vi "Confocal_0823.vi"() -> ()   [LabVIEW 2017]
uses:
  <vilib>/Math Plots/2D Math Plots/XY Plot Matrix/XY Plot Matrix XCtrl/XY Plot Matrix.xctl
  Public/Documents/SIToolkit/LabVIEW/ExamplesXX_4_3_1_4/Spectroscopy Applications/GlobalCamOpen.vi
  Public/Documents/SIToolkit/LabVIEW/ExamplesXX_4_3_1_4/Spectroscopy Applications/GlobalInitializeFlag.vi
  Public/Documents/SIToolkit/LabVIEW/ExamplesXX_4_3_1_4/Spectroscopy Applications/GlobalTimingMode.vi
  Public/Documents/SIToolkit/LabVIEW/ExamplesXX_4_3_1_4/Spectroscopy Applications/GlobalFramesToStr.vi
  Public/Documents/SIToolkit/LabVIEW/ExamplesXX_4_3_1_4/Spectroscopy Applications/GlobalAcquireFocusFlag.vi
  Public/Documents/SIToolkit/LabVIEW/ExamplesXX_4_3_1_4/Spectroscopy Applications/GlobalExposure.vi
  <vilib>/Math Plots/2D Math Plots/XY Plot Matrix/XY Plot Matrix Datatype/XY Plot Matrix Datatype.lvclass
panel:
  out "Position 7":dbl[](array[numeric]) format="%.6f"
  out "Position 4":dbl[](array[numeric]) format="%.6f"
  in  "error PI Stage":errorcluster
  out "error out 2":errorcluster
  in  "Tab Control":T1(tab)
  in  "Focus/Acquire Mode":u32=1 min=1 max=5 step=1
  in  "Number of Frames to store":u32=1 min=1 step=1
  in  "Timing Mode":u32(ring)=1 items=["N/A", "Free Run/Timed", "Trigger First (PM only)", "Ext Sync/Strobed ", "Variable Exp (PM only)", "Flash Mode (PM only)"]
  out "Pixel Time":i32
  out "Bit Depth":i32
  out "ReadOut port":i32
  out "ADC Speed":i32
  in  "Set Experiment \nParameters, Initialize \nCamera/Controller":bool
  out "Read Temp.":dbl format="%.2f"
  in  "Set Temp.":dbl format="%.2f"
  in  "Exposure 2":dbl=0.2 format="%.2f"
  out "Controller Initialized":bool
  in  "error in":errorcluster
  out "error out":errorcluster
  in  "Power":dbl=10.0
  in  "Frequency":dbl=2810.0
  in  "Release Camera":bool
  out "Position 6":dbl[](array[numeric]) format="%.6f"
  out "Conn. Axis 5":string[](array[string])
  out "error out 3":errorcluster
  out "COM Error":bool
  out "Camera Opened":bool
  in  "Number of Steps Left":dbl=5.0 format="%#_13g"
  in  "OK Button 5":bool
  in  "Step Size (microns)":dbl[](array[numeric])=[0.01]
  out "XY Plot Matrix":refnum<class "XY Plot Matrix Datatype.lvclass">[](xcontrol)
  in  "Number of Steps Down":dbl=5.0 format="%#_13g"
  out "Position":dbl[](array[numeric]) format="%.6f"
  out "Position 3":dbl[](array[numeric]) format="%.6f"
  in  "stop 2":bool
  out "Line Number":i32
  out "Position 2":dbl[](array[numeric]) format="%.6f"
  in  "?":bool
  out "Position 5":dbl[](array[numeric]) format="%.6f"
  in  "Step Size (microns) Y":dbl[](array[numeric])=[0.01]
  in  "Step Size (microns) X":dbl[](array[numeric])=[0.01]
  out "Position 8":dbl[](array[numeric]) format="%.6f"
  in  "?":bool
  out "Acquire Graph":sgl[](graph)
  out "Collecting Data":bool
  in  "Full File Name for Acqure":path
  in  "OK Button":bool
  # "The following are read \nfrom camera after setting\nvalues to left.\n-1 value means item is not \nsupported by camera."
  # "Stage position on connection."
  # "Be sure to put in a full file name below before starting."
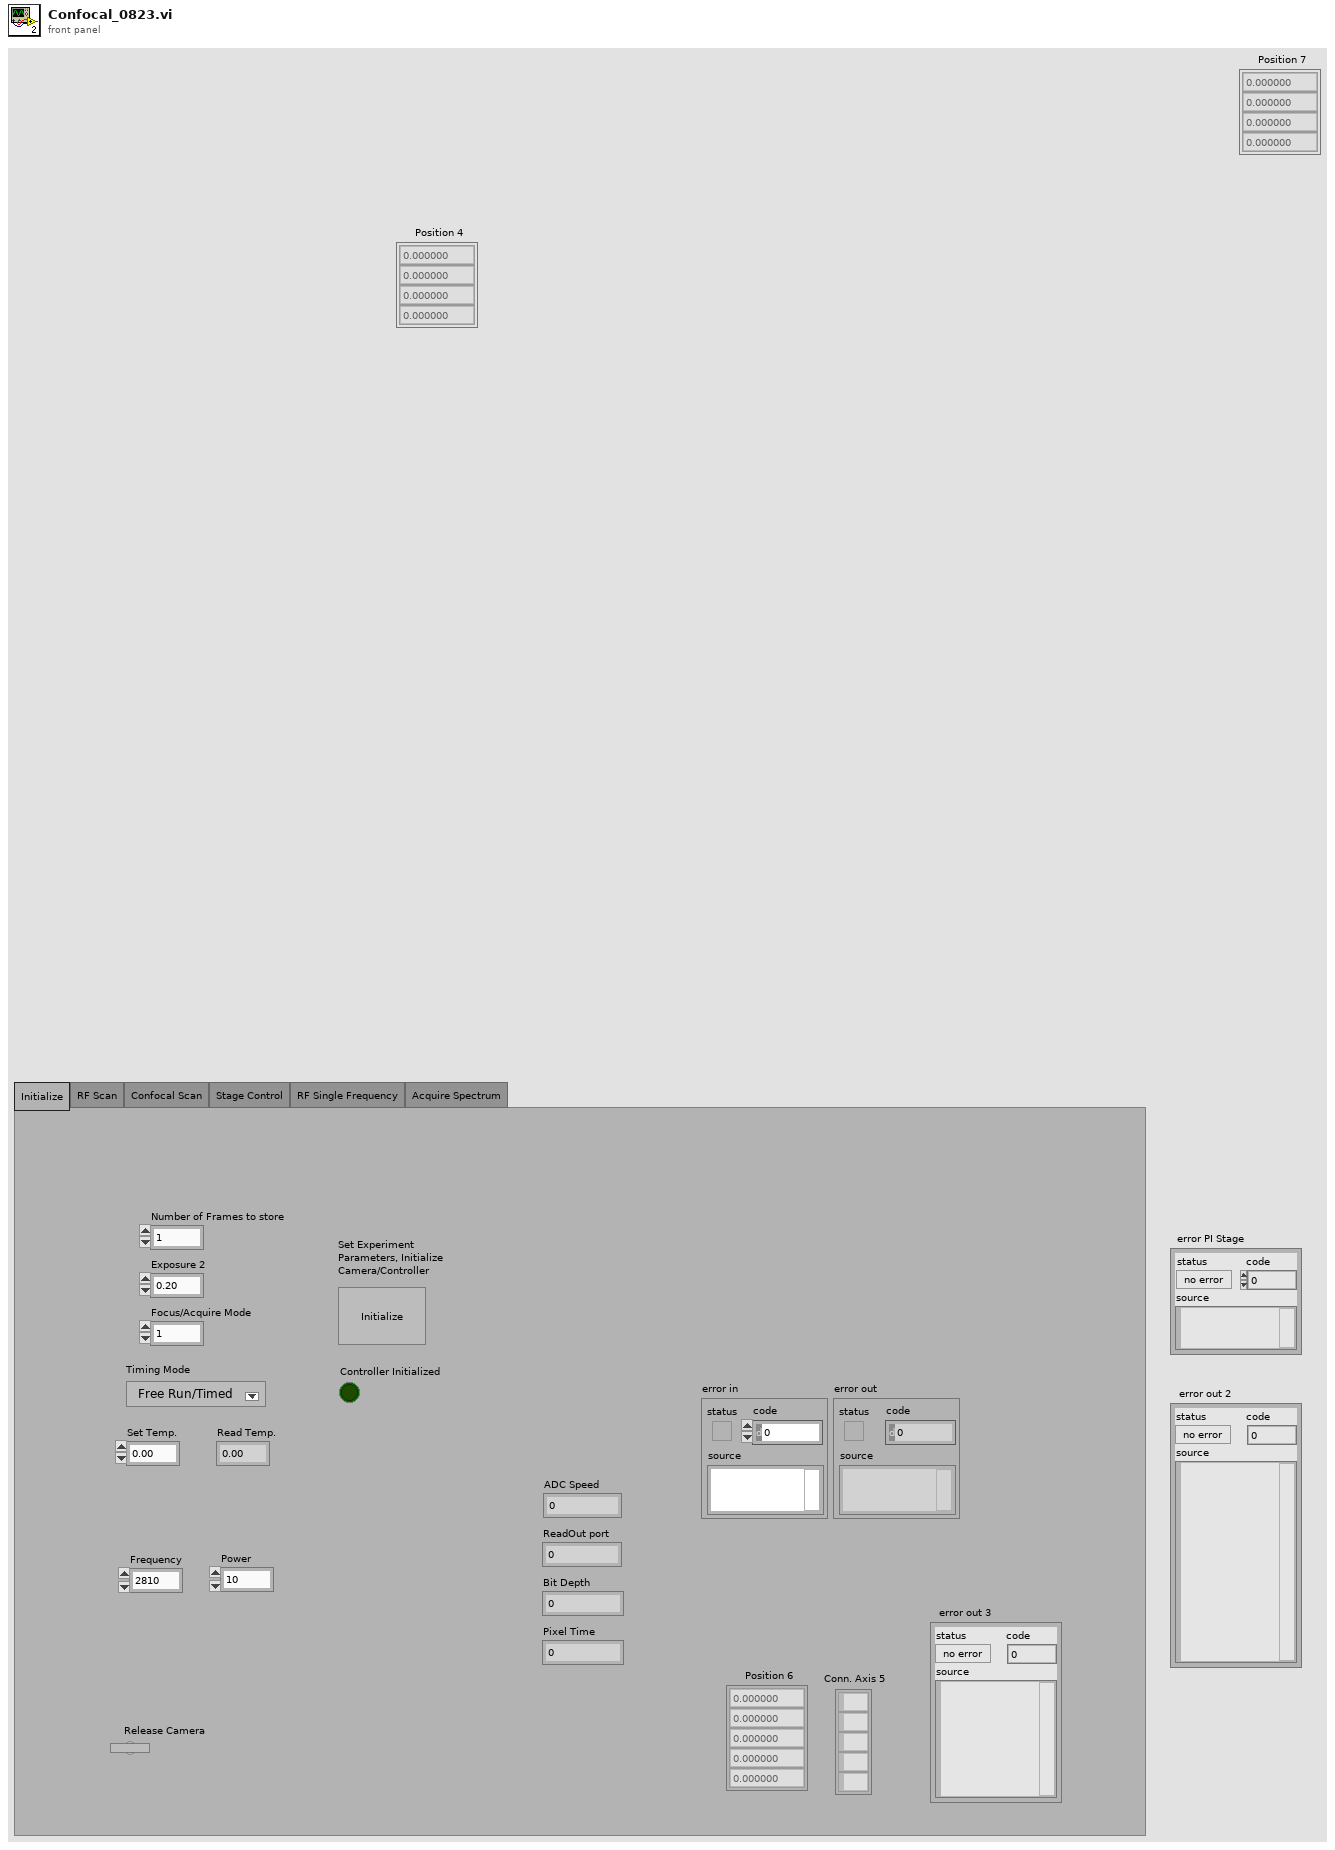
[diagram p1: front panel]
types:
  T1 = enum32{"Initialize", "RF Scan", "Confocal Scan", "Stage Control", "RF Single Frequency", "Acquire Spectrum"}
  T2 = cluster{"X start":u32, "X end":u32, "X Binning/Grouping":u32, "Y start":u32, "Y end":u32, "Y Binning/Grouping":u32}
  T3 = cluster{"Host address/name":string, "Port":i32, "Board":i32, "TCP/IP Search?":bool}
  T4 = cluster{"Camera Handle":u32, "Pulser Handle":u32, "File Handle":u32, "Display Handle":u32, "Image Handle":u32}
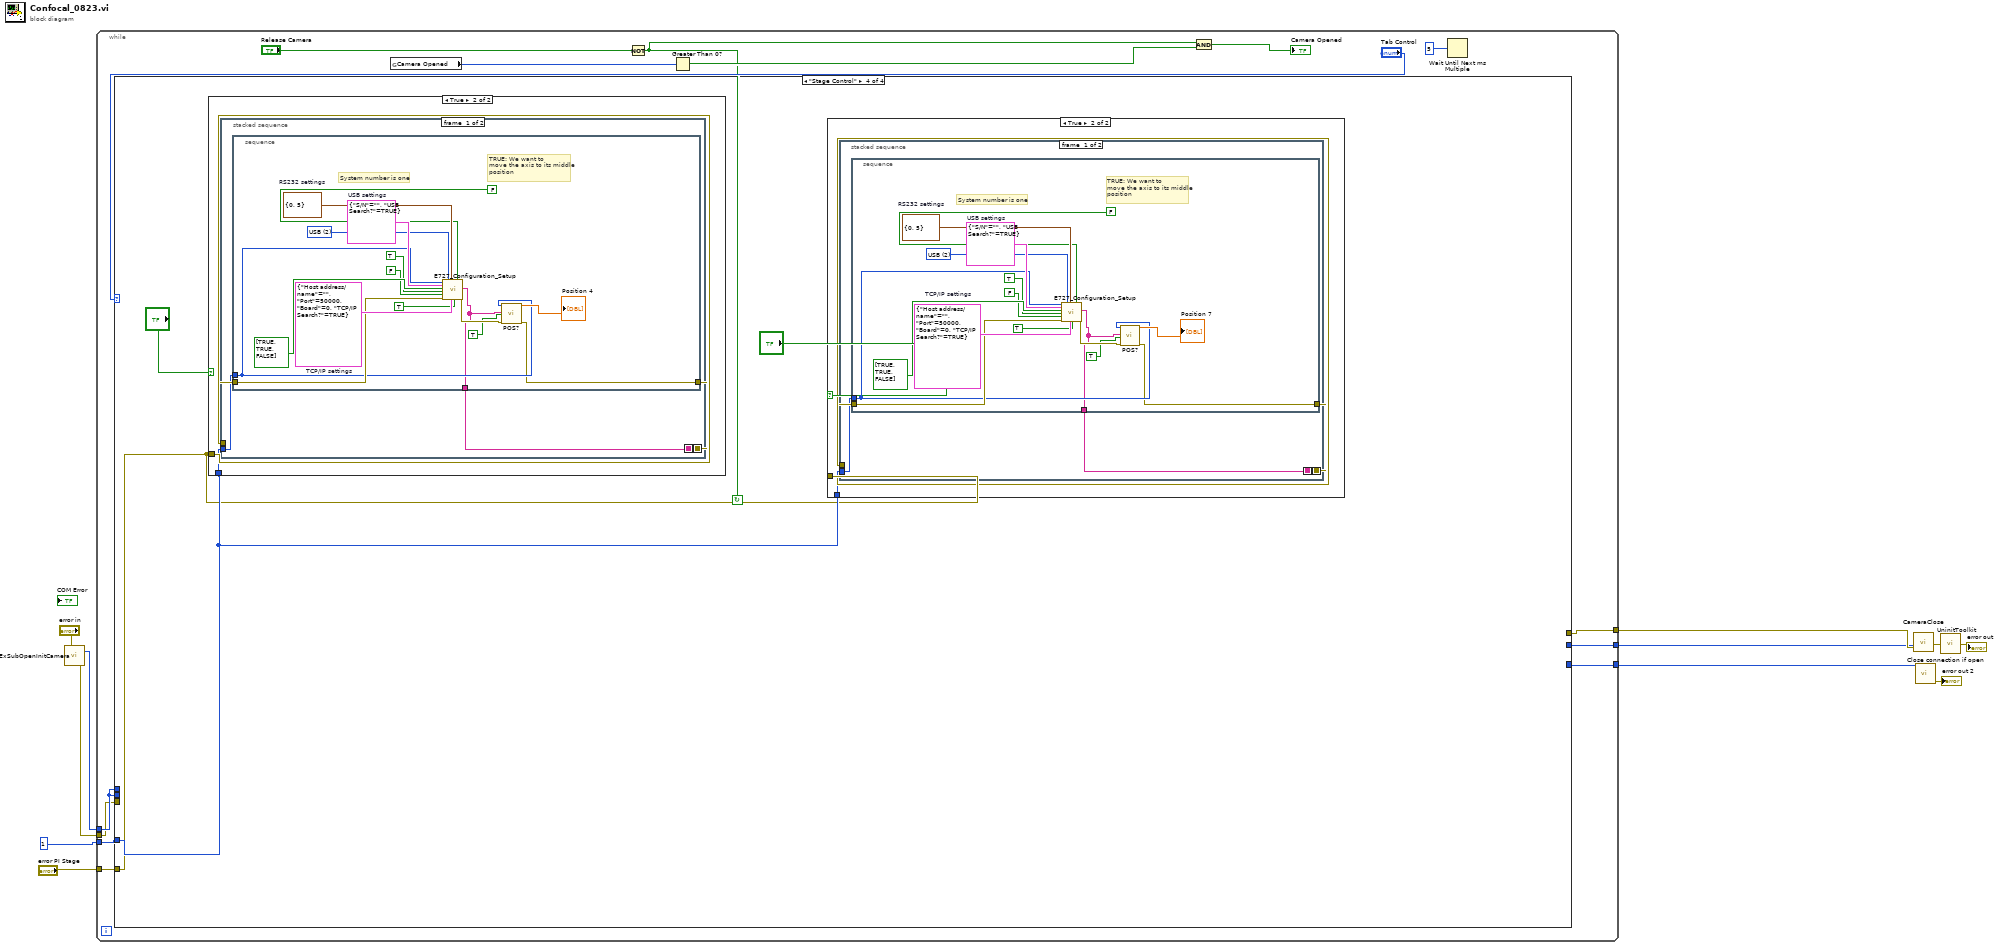
[diagram p0: block diagram]
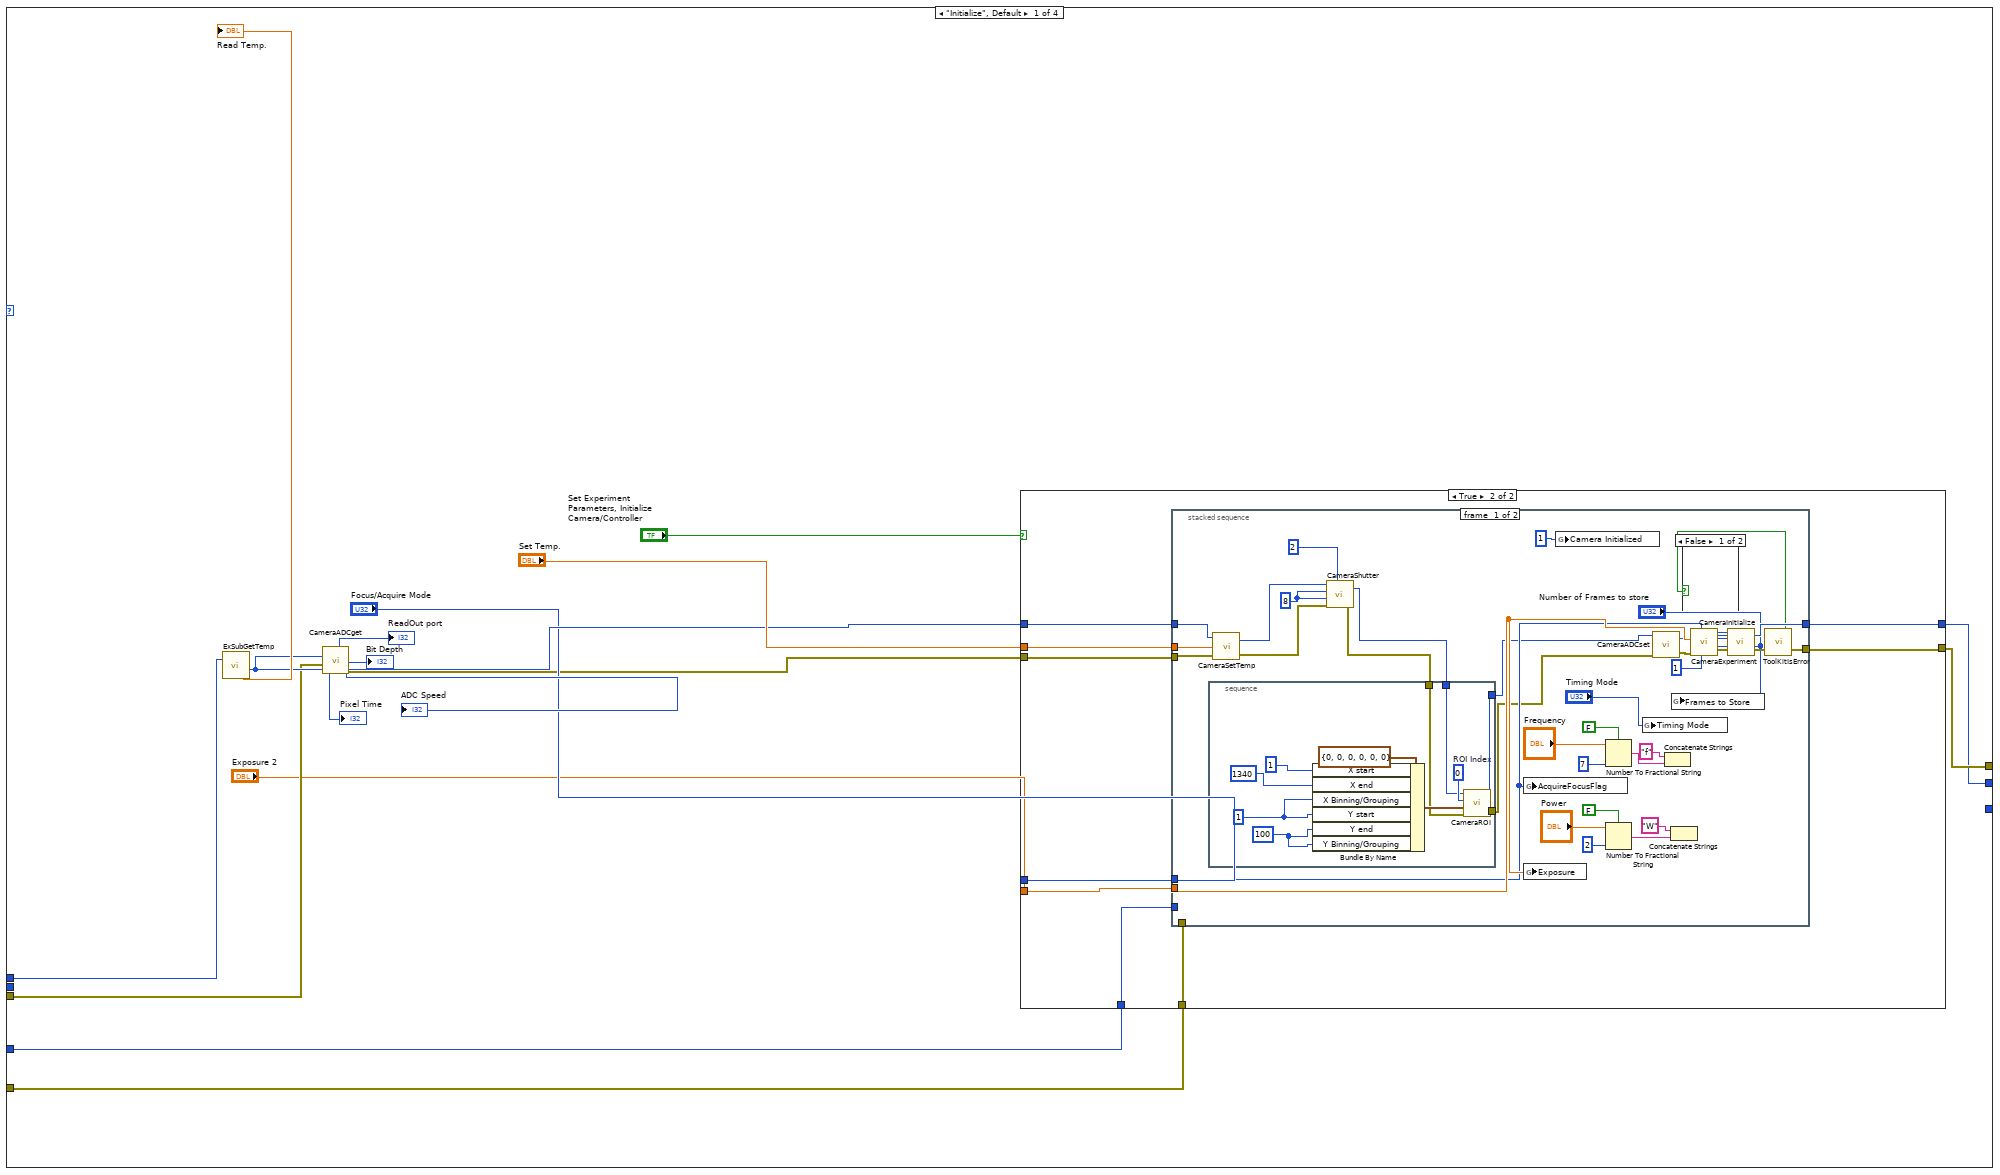
[diagram p2: hidden frame]
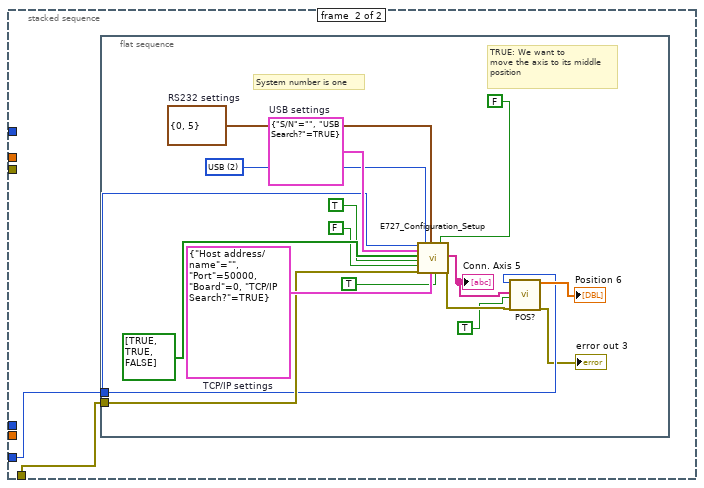
[diagram p5: hidden frame]
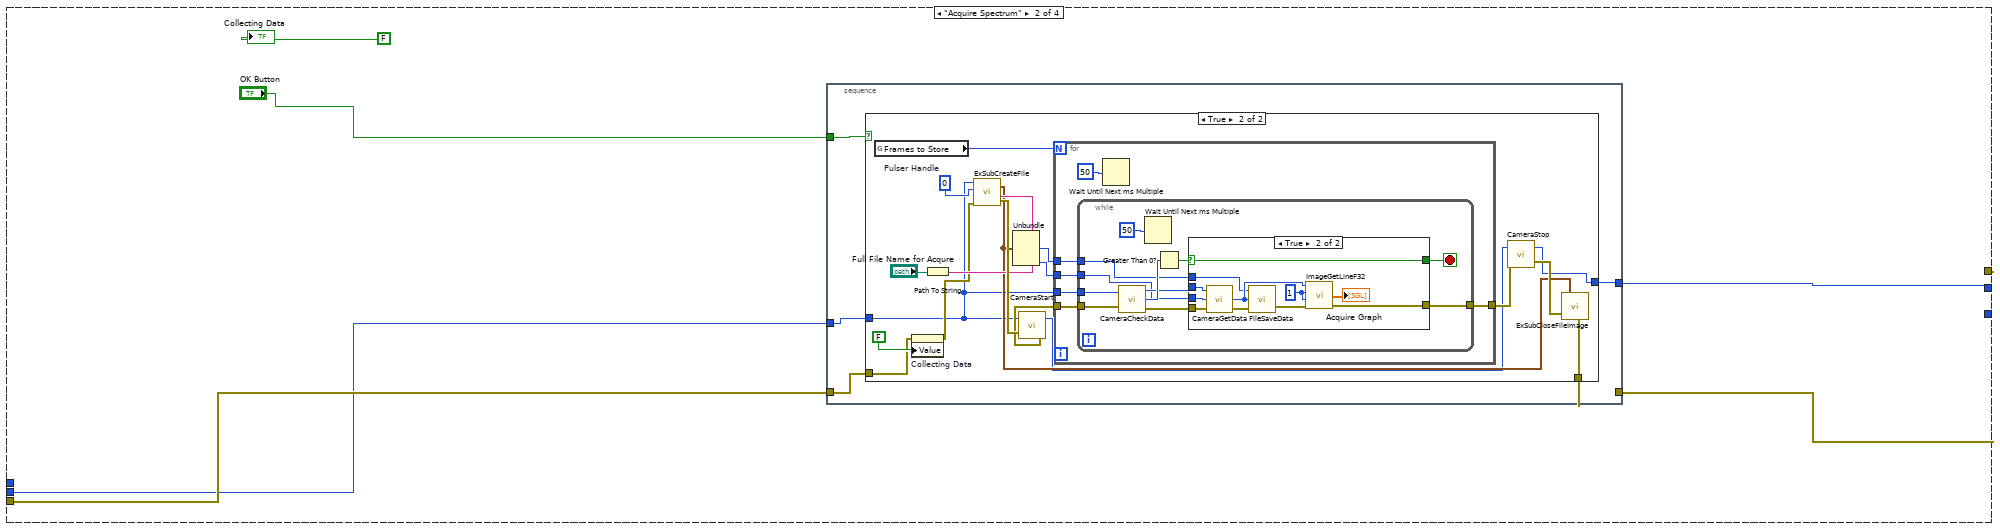
[diagram p6: hidden frame]
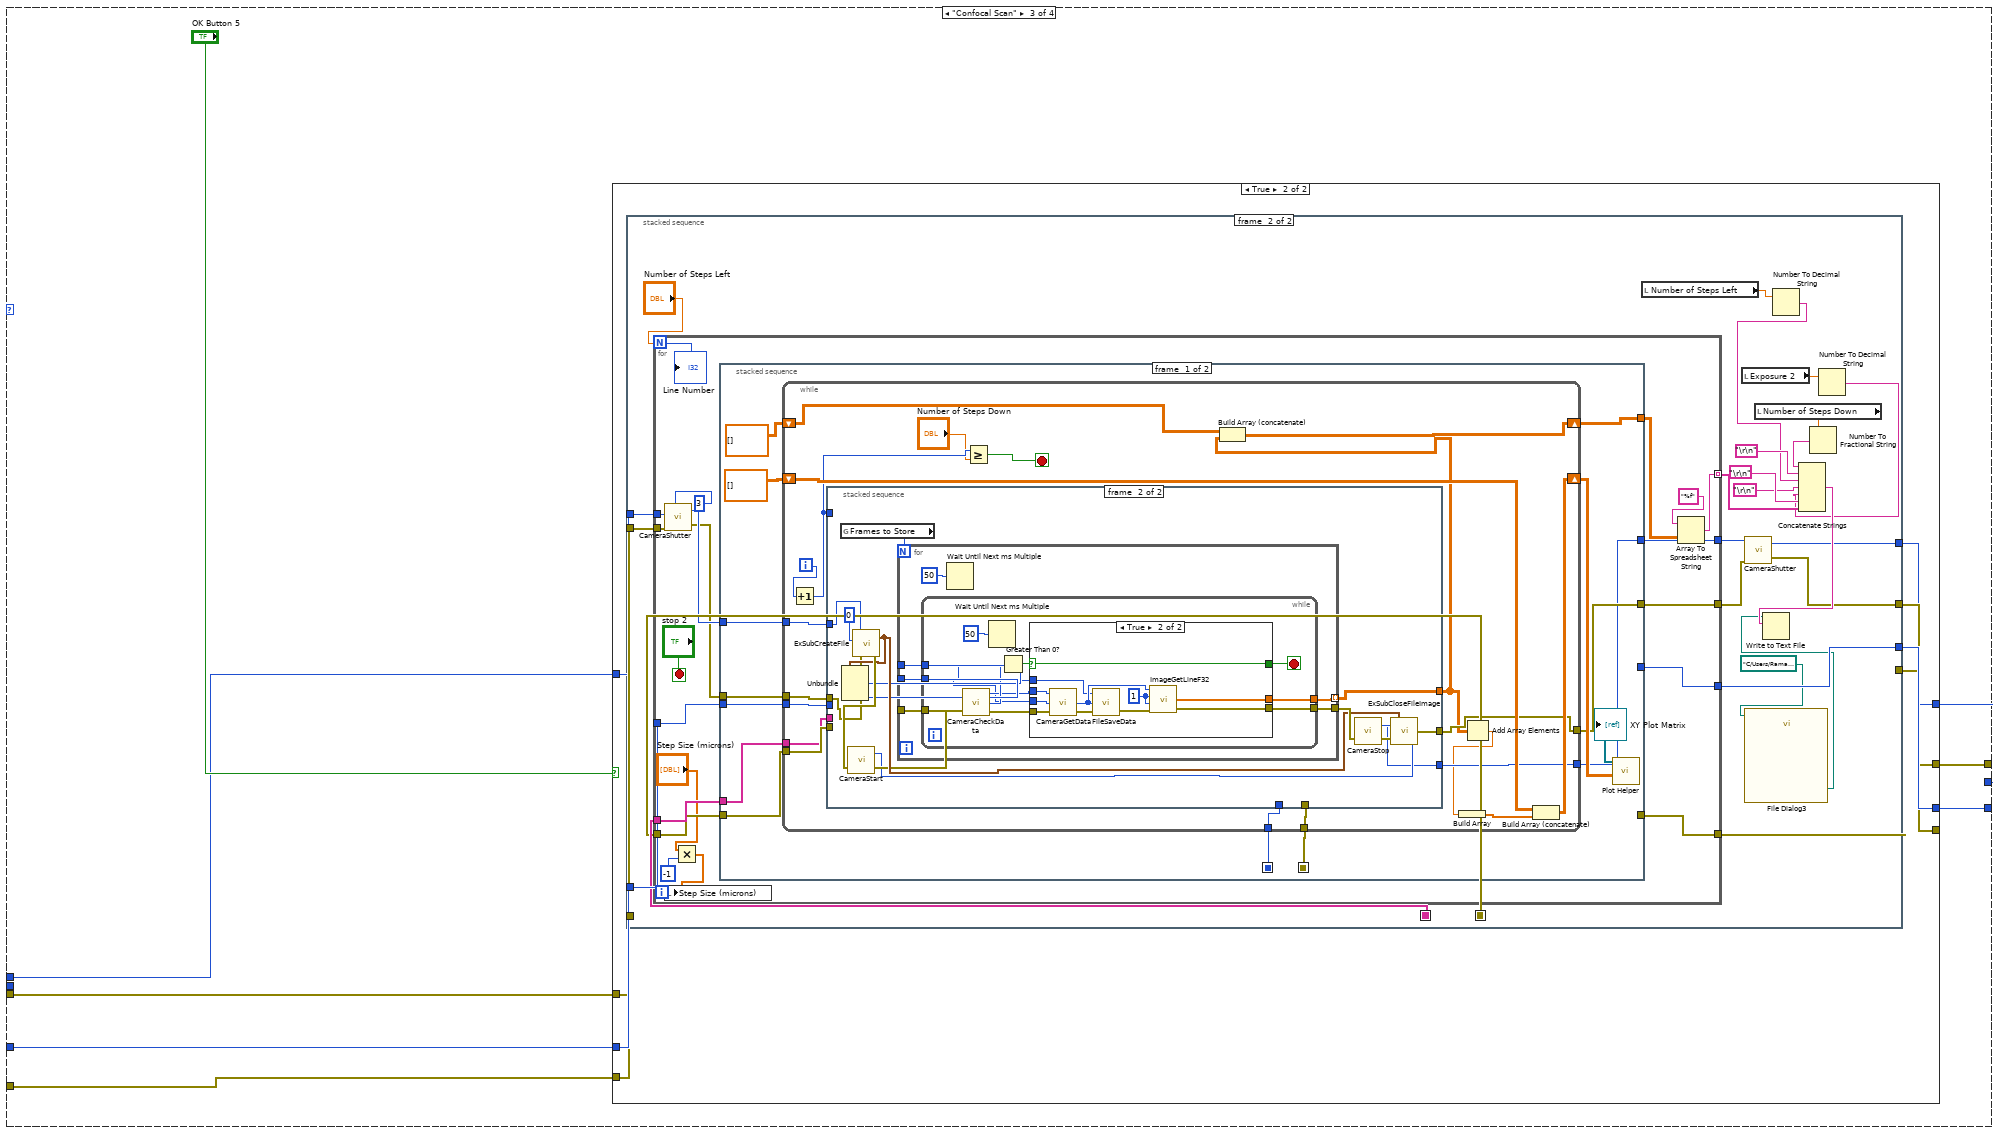
[diagram p9: hidden frame]
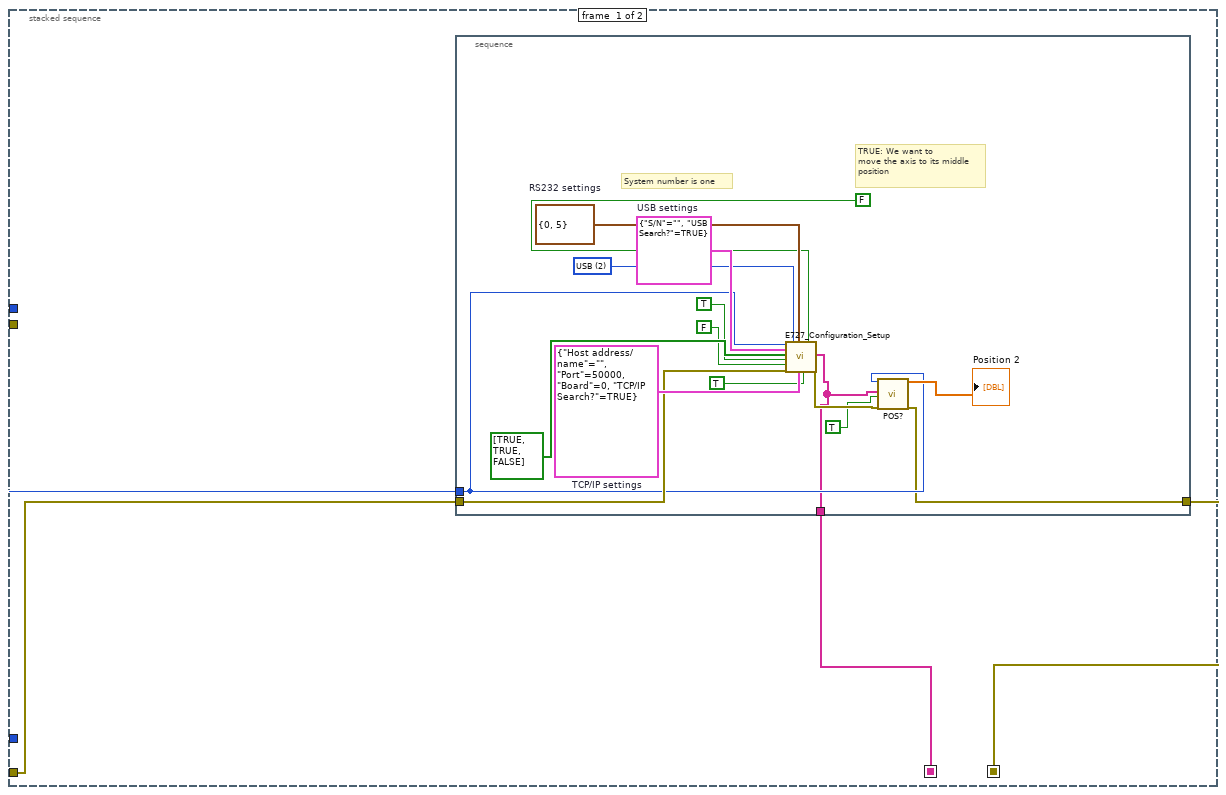
[diagram p11: hidden frame]
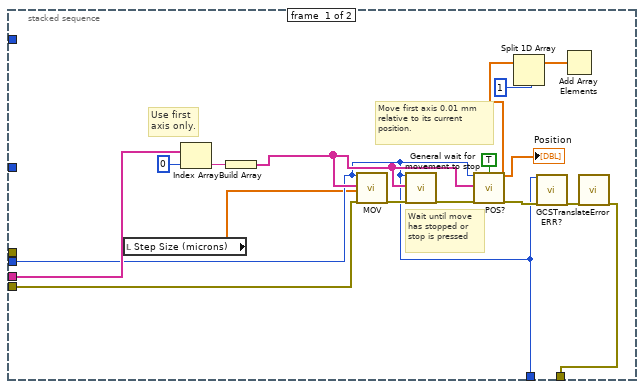
[diagram p12: hidden frame]
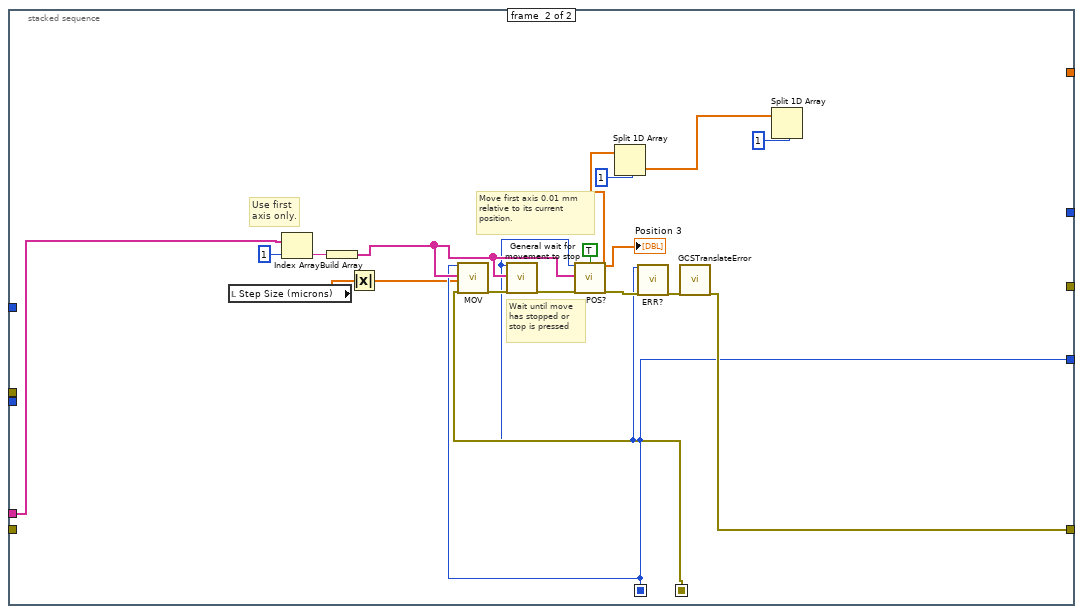
[diagram p14: hidden frame]
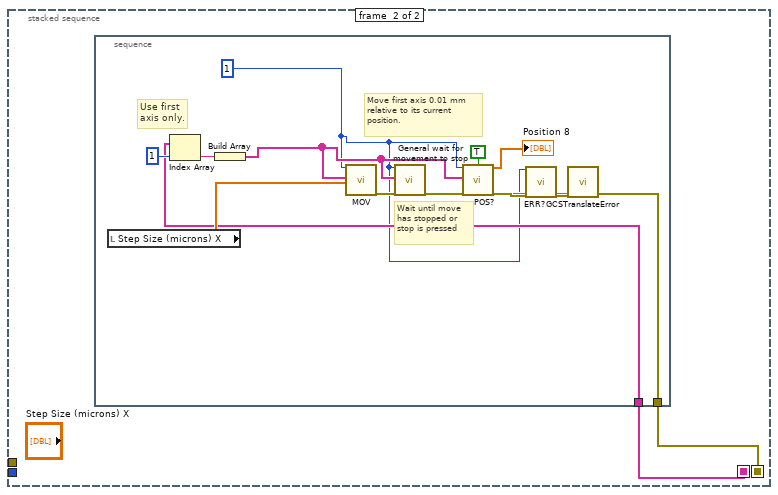
[diagram p16: hidden frame]
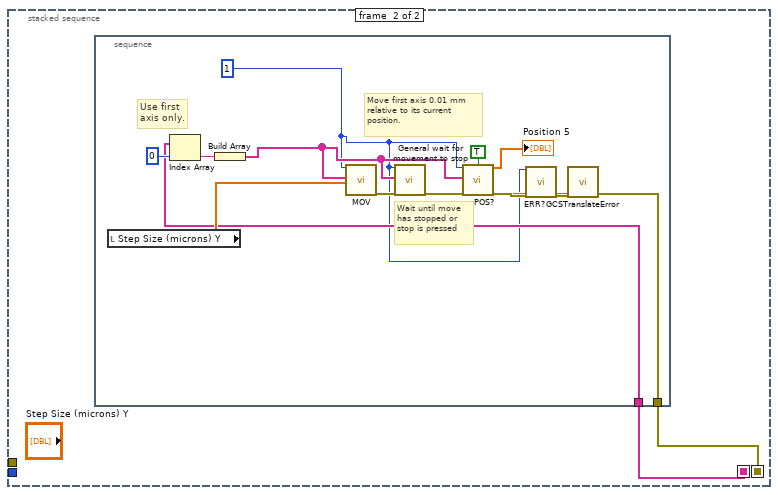
[diagram p18: hidden frame]
diagram:
  n1 = call "ExSubOpenInitCamera.vi"("error in (no error)"="error in") -> ("Camera Handle"=w10:u32, "error out"=w9:errorcluster)
  n2 = while {
    tunnel: w10 -> [w19]
    tunnel: w9 -> [w18]
    tunnel: [w17] -> w8
    tunnel: [w15] -> w5
    tunnel: "error PI Stage" -> [w14]
    tunnel: 1 -> [w12]
    tunnel: [w13] -> w1
    stop <- w16 continue-if-true
    n3 = case shown="\"Stage Control\"" "Tab Control" {
      tunnel: w19 -> [w34 _ w181 _]
      tunnel: w19 -> [_ w123 _ _]
      tunnel: w18 -> [w33 w124 w182 _]
      tunnel: [w28 w120 w183 _] -> w15
      tunnel: [w30 w121 w184 _] -> w17
      tunnel: w14 -> [w26 _ w186 w375]
      tunnel: w12 -> [w27 _ w188 w376]
      tunnel: [_ _ w187 _] -> w13
      frame "Initialize", Default {
        n4 = call "ExSubGetTemp.vi"("Camera Handle"=w34) -> ("Camera Handle"=w39:u32, "Temperature Real"=→"Read Temp.":dbl)  [unwired: 1 in, 1 out]
        n5 = call <userlib>:"CameraADCget.vi"("Camera handle"=w39, "error in (no error)"=w33) -> ("Bit Depth"=→"Bit Depth":i32, "Pixel Time"=→"Pixel Time":i32, "Readout Port"=→"ReadOut port":i32, "ADC Speed"=→"ADC Speed":i32, "error out"=w32:errorcluster)  [unwired: 3 out]
        n6 = case shown="True" "Set Experiment \nParameters, Initialize \nCamera/Controller" {
          tunnel: "Exposure 2" -> [_ w53]
          tunnel: "Set Temp." -> [_ w54]
          tunnel: w39 -> [w46 w55]
          tunnel: [w46 w52] -> w28
          tunnel: "Focus/Acquire Mode" -> [_ w51]
          tunnel: w32 -> [w45 w50]
          tunnel: [w45 w49] -> w30
          tunnel: w27 -> [_ w48]
          tunnel: w26 -> [_ w47]
          frame False {
          }
          frame True {
            n7 = stacked-sequence {
              tunnel: w55 -> [w90 _]
              tunnel: w54 -> [w89 _]
              tunnel: w53 -> [w88 _]
              tunnel: [w87 _] -> w52
              tunnel: w51 -> [w86 _]
              tunnel: w50 -> [w85 _]
              tunnel: [w84 _] -> w49
              tunnel: w48 -> [_ w102]
              tunnel: w47 -> [_ w103]
              frame #0 {
                w56 = 8
                n8 = call <userlib>:"CameraSetTemp.vi"("error in (no error)"=w85, "Temperature"=w89, "Camera Handle"=w90) -> ("error out"=w59:errorcluster, "Camera Handle"=w61:u32)
                n9 = call <userlib>:"CameraShutter.vi"("Camera Handle"=w61, "Shutter Comp Time: Pre Open"=w56, "Shutter Comp Time: Post Open"=w56, "error in"=w59, "Shutter State"=2) -> ("Camera Handle"=w60:u32, "error out"=w58:errorcluster)
                n10 = stacked-sequence {
                  tunnel: [w98] -> w63
                  tunnel: w60 -> [w95]
                  tunnel: w58 -> [w94]
                  tunnel: [w93] -> w62
                  frame #0 {
                    w97 = 100
                    w91 = 1
                    w100 = u32 0  # ROI Index
                    n11 = Bundle By Name(cluster=T2 {"X start"=0, "X end"=0, "X Binning/Grouping"=0, "Y start"=0, "Y end"=0, "Y Binning/Grouping"=0} ("ROI Params"), "X start"=1, "X end"=1340, "X Binning/Grouping"=w91, "Y start"=w91, "Y end"=w97, "Y Binning/Grouping"=w97) -> (w101:T2)
                    n12 = call <userlib>:"CameraROI.vi"("error in"=w94, "ROI Params"=w101, "ROI Index"=w100, "Camera Handle"=w95) -> ("error out"=w93:errorcluster, "Camera Handle"=w98:u32)
                  }
                }
                n13 = global write "GlobalAcquireFocusFlag.vi" "AcquireFocusFlag"(w86) -> ()
                n14 = global write "GlobalExposure.vi" "Exposure"(w88) -> ()
                n15 = global write "GlobalInitializeFlag.vi" "Camera Initialized"(1) -> ()
                n16 = Number To Fractional String(use system decimal point (T)=FALSE, number="Frequency", precision (6)=7) -> (F-format string=w65:string)  [unwired: 1 in]
                n17 = Number To Fractional String(use system decimal point (T)=FALSE, number="Power", precision (6)=2) -> (F-format string=w72:string)  [unwired: 1 in]
                n18 = global write "GlobalTimingMode.vi" "Timing Mode"("Timing Mode") -> ()
                n19 = call <userlib>:"CameraADCset.vi"("error in (no error)"=w62, "Camera Handle"=w63) -> ("error out"=w80:errorcluster, "Camera Handle"=w79:u32)  [unwired: 4 in]
                n20 = Concatenate Strings("f", w65) -> ()  [unwired: 1 out]
                n21 = Concatenate Strings("W", w72) -> ()  [unwired: 1 out]
                n22 = global write "GlobalFramesToStr.vi" "Frames to Store"("Number of Frames to store") -> ()
                n23 = call <userlib>:"CameraExperiment.vi"("Number of Accumulations"=1, "Acquire / Focus Flag"=w86, "error in"=w80, "Number of Images"="Number of Frames to store", "Exposure (sec)"=w88, "Camera Handle"=w79) -> ("error out"=w78:errorcluster, "Camera Handle"=w77:u32)
                n24 = call <userlib>:"CameraInitialize.vi"("error in"=w78, "Camera Handle"=w77) -> ("error out"=w75:errorcluster, "Camera Handle"=w87:u32)
                n25 = call <userlib>:"ToolKitIsError.vi"("error in"=w75) -> ("error out"=w84:errorcluster, "Error Flag"=w76:bool)  [unwired: 1 in]
                n26 = case shown="False" w76 {
                  frame False {
                  }
                  frame True {
                  }
                }
              }
              frame #1 {
                n27 = flat-sequence {
                  tunnel: w103 -> [w107]
                  tunnel: w102 -> [w106]
                  frame #0 {
                    w119 = cluster{"S/N":string, "USB Search?":bool} {"S/N"="", "USB Search?"=TRUE}  # USB settings
                    w115 = u16 2 items=["RS232", "TCP/IP", "USB"] ("Interface")
                    w114 = cluster{"Portnumber":i32, "Baudrate":u16} {"Portnumber"=0, "Baudrate"=5}  # RS232 settings
                    w113 = T3 {"Host address/name"="", "Port"=50000, "Board"=0, "TCP/IP Search?"=TRUE}  # TCP/IP settings
                    # "TRUE: We want to\nmove the axis to its middle\nposition"
                    # "System number is one"
                    n28 = call "E727_Configuration_Setup.vi"("System no."=w106, "USB settings"=w119, "Are stages connected?"=bool[] [TRUE, TRUE, FALSE], "Change servo status to ON?"=TRUE ("Use dialog to define\nconnected stages?"), "Perform autozero?"=FALSE ("Use dialog to define\nconnected stages?"), "error in"=w107, "Interface"=w115, "RS232 settings"=w114, "TCP/IP settings"=w113, "Stop wave generator\noutput (if any)"=TRUE ("All axes?"), "Move to middle?"=FALSE) -> ("All conn. axes"=w105:string[], "error out"=w109:errorcluster)  [unwired: 3 in, 4 out]
                    "Conn. Axis 5" <- w105
                    n29 = call "POS?.vi"("System no."=w106, "Axes to query"=w105, "All axes?"=TRUE, "error in"=w109) -> ("Position"=→"Position 6":dbl[], "error out"=→"error out 3":errorcluster)  [unwired: 1 in, 13 out]
                  }
                }
              }
            }
          }
        }
        n30 = global read "GlobalInitializeFlag.vi" "Camera Initialized"() -> (w42:u32)
        n31 = Greater Than 0?(x=w42) -> (x > 0?=→"Controller Initialized":bool)
      }
      frame "Acquire Spectrum" {
        n32 = stacked-sequence {
          tunnel: [w127] -> w121
          tunnel: [w128] -> w120
          tunnel: w124 -> [w130]
          tunnel: "OK Button" -> [w129]
          tunnel: w123 -> [w126]
          frame #0 {
            n33 = case shown="True" w129 {
              tunnel: [w131 w143] -> w128
              tunnel: [w132 w135] -> w127
              tunnel: w130 -> [w132 w134]
              tunnel: w126 -> [w131 w133]
              frame False {
              }
              frame True {
                w137 = u32 0  # Pulser Handle
                n34 = global read "GlobalFramesToStr.vi" "Frames to Store"() -> (w146:u32)
                n35 = property on="Collecting Data" class="Bool (strict)"(error in=w134, "Value"=FALSE) -> (error out=w145:errorcluster)  [unwired: 1 in, 1 out]
                n36 = Path To String(path="Full File Name for Acqure") -> (string=w148:string)
                n37 = call "ExSubCreateFile.vi"("error in (no error)"=w145, "File and Display Name"=w148, "Pulser Handle"=w137, "Camera Handle"=w133) -> ("error out"=w150:errorcluster, "Handles Out"=w141:T4)
                n38 = Unbundle(w141) -> ("File Handle"=w136:u32, "Image Handle"=w139:u32)  [unwired: 3 out]
                n39 = call <userlib>:"CameraStart.vi"("error in"=w150, "Camera Handle"=w133) -> ("error out"=w140:errorcluster, "Camera Handle"=w138:u32)
                n40 = for {
                  N: w146 -> [_]
                  tunnel: w133 -> [w155]
                  tunnel: w140 -> [w154]
                  tunnel: [w153] -> w142
                  tunnel: w136 -> [w152]
                  tunnel: w139 -> [w151]
                  n41 = while {
                    tunnel: [w162] -> w153
                    tunnel: w155 -> [w160]
                    tunnel: w154 -> [w159]
                    tunnel: w152 -> [w158]
                    tunnel: w151 -> [w157]
                    stop <- w163 stop-if-true
                    n42 = call <userlib>:"CameraCheckData.vi"("Camera Handle"=w160, "error in"=w159) -> ("Camera Handle"=w165:u32, "Number Of Frames Available"=w167:i32, "error out"=w164:errorcluster)
                    n43 = Wait Until Next ms Multiple(millisecond multiple=u32 50) -> ()  [unwired: 1 out]
                    n44 = Greater Than 0?(x=w167) -> (x > 0?=w166:bool)
                    n45 = case shown="True" w166 {
                      selector: w166 -> [w168 w178]
                      tunnel: w165 -> [_ w180]
                      tunnel: w164 -> [w169 w179]
                      tunnel: [w168 w178] -> w163
                      tunnel: [w169 w173] -> w162
                      tunnel: w158 -> [_ w171]
                      tunnel: w157 -> [_ w170]
                      frame False {
                      }
                      frame True {
                        w174 = 1
                        n46 = call <userlib>:"CameraGetData.vi"("error in"=w179, "Image/Data Handle"=w170, "Camera Handle"=w180) -> ("error out"=w177:errorcluster, "Image/Data Handle"=w175:u32)  [unwired: 1 out]
                        n47 = call <userlib>:"FileSaveData.vi"("error in"=w177, "Image Handle"=w175, "File Handle"=w171) -> ("error out"=w176:errorcluster)  [unwired: 1 out]
                        n48 = call <userlib>:"ImageGetLineF32.vi"("error in"=w176, "Z Position"=w174, "Y Position"=w174, "Data Handle"=w175) -> ("error out"=w173:errorcluster, "Array F32"=→"Acquire Graph":sgl[])  [unwired: 1 out]
                      }
                    }
                  }
                  n49 = Wait Until Next ms Multiple(millisecond multiple=u32 50) -> ()  [unwired: 1 out]
                }
                n50 = call <userlib>:"CameraStop.vi"("error in"=w142, "Camera Handle"=w138) -> ("error out"=w147:errorcluster, "Camera Handle"=w143:u32)
                n51 = call "ExSubCloseFileImage.vi"("error in (no error)"=w147, "Handles In"=w141) -> ("error out"=w135:errorcluster)
              }
            }
          }
        }
        "Collecting Data" <- FALSE
      }
      frame "Confocal Scan" {
        n52 = case shown="True" "OK Button 5" {
          tunnel: w188 -> [_ w196]
          tunnel: [_ w195] -> w187
          tunnel: [_ w194] -> _
          tunnel: w186 -> [_ w193]
          tunnel: [_ w192] -> w184
          tunnel: [_ w191] -> w183
          tunnel: w182 -> [_ w190]
          tunnel: w181 -> [_ w189]
          frame False {
          }
          frame True {
            n53 = stacked-sequence {
              seq-local: [w198 _] -> [_ w238]
              seq-local: [w197 _] -> [_ w237]
              tunnel: w196 -> [w199 w241]
              tunnel: [_ w240] -> w195
              tunnel: [_ w239] -> w194
              tunnel: w193 -> [w200 _]
              tunnel: [_ w230] -> w192
              tunnel: [_ w232] -> w191
              tunnel: w190 -> [_ w229]
              tunnel: w189 -> [_ w228]
              frame #0 {
                n54 = stacked-sequence {
                  tunnel: w200 -> [w204]
                  tunnel: w199 -> [w203]
                  tunnel: [w202] -> w197
                  tunnel: [w201] -> w198
                  frame #0 {
                    w216 = cluster{"S/N":string, "USB Search?":bool} {"S/N"="", "USB Search?"=TRUE}  # USB settings
                    w212 = u16 2 items=["RS232", "TCP/IP", "USB"] ("Interface")
                    w211 = cluster{"Portnumber":i32, "Baudrate":u16} {"Portnumber"=0, "Baudrate"=5}  # RS232 settings
                    w210 = T3 {"Host address/name"="", "Port"=50000, "Board"=0, "TCP/IP Search?"=TRUE}  # TCP/IP settings
                    # "TRUE: We want to\nmove the axis to its middle\nposition"
                    # "System number is one"
                    n55 = call "E727_Configuration_Setup.vi"("System no."=w203, "USB settings"=w216, "Are stages connected?"=bool[] [TRUE, TRUE, FALSE], "Change servo status to ON?"=TRUE ("Use dialog to define\nconnected stages?"), "Perform autozero?"=FALSE ("Use dialog to define\nconnected stages?"), "error in"=w204, "Interface"=w212, "RS232 settings"=w211, "TCP/IP settings"=w210, "Stop wave generator\noutput (if any)"=TRUE ("All axes?"), "Move to middle?"=FALSE) -> ("All conn. axes"=w201:string[], "error out"=w206:errorcluster)  [unwired: 3 in, 4 out]
                    n56 = call "POS?.vi"("System no."=w203, "Axes to query"=w201, "All axes?"=TRUE, "error in"=w206) -> ("Position"=→"Position 2":dbl[], "error out"=w202:errorcluster)  [unwired: 1 in, 13 out]
                  }
                }
              }
              frame #1 {
                n57 = for {
                  N: "Number of Steps Left" -> [w242]
                  tunnel: w241 -> [w258]
                  tunnel: [w252] -> w227 mode=indexing
                  tunnel: [w260] -> w239
                  tunnel: w238 -> [w259]
                  tunnel: w237 -> [w257]
                  tunnel: [w256] -> w240
                  tunnel: [w249] -> w231
                  tunnel: [w248] -> w233
                  tunnel: w229 -> [w244]
                  tunnel: w228 -> [w243]
                  stop <- "stop 2" stop-if-true
                  n58 = call <userlib>:"CameraShutter.vi"("Shutter Comp Time: Pre Open"=w243, "error in"=w244, "Shutter State"=3) -> ("Camera Handle"=w246:u32, "error out"=w245:errorcluster)  [unwired: 2 in]
                  n59 = Multiply(x="Step Size (microns)", y=-1) -> (x*y=w253:dbl[])
                  n60 = local write "Step Size (microns)"(w253) -> ()
                  n61 = stacked-sequence {
                    seq-local: [w267 _] -> [_ w361]
                    seq-local: [w268 _] -> [_ w363]
                    tunnel: [_ w362] -> w260
                    tunnel: w259 -> [w271 w364]
                    tunnel: w258 -> [w269 _]
                    tunnel: w257 -> [w270 _]
                    tunnel: [_ w361] -> w256
                    tunnel: [w266 _] -> w250
                    tunnel: [w265 _] -> w249
                    tunnel: [w264 _] -> w248
                    tunnel: w246 -> [w263 _]
                    tunnel: w245 -> [w262 _]
                    frame #0 {
                      n62 = while {
                        shift-right: [w293] -> w272
                        shift-left: dbl[][] [] -> [w294]
                        shift-right: [w276] -> w266
                        shift-left: dbl[][] [] -> [w277]
                        tunnel: w270 -> [w292]
                        tunnel: w271 -> [w291]
                        tunnel: w269 -> [w288]
                        tunnel: [w287] -> w268
                        tunnel: [w286] -> w267
                        tunnel: [w283] -> w265
                        tunnel: [w282] -> w264
                        tunnel: w263 -> [w281]
                        tunnel: w262 -> [w280]
                        i -> [w289]
                        stop <- w290 stop-if-true
                        n63 = Increment(x=w289) -> (x+1=w285:i32)
                        n64 = stacked-sequence {
                          tunnel: w292 -> [w311 _]
                          tunnel: [w304 _] -> w287
                          tunnel: w291 -> [w302 _]
                          tunnel: w285 -> [_ _]
                          tunnel: w288 -> [w297 _]
                          tunnel: [w297 _] -> w286
                          tunnel: [_ w316] -> w278
                          tunnel: [_ w315] -> w283
                          tunnel: [_ w314] -> w282
                          tunnel: w281 -> [_ w313]
                          tunnel: w280 -> [_ w312]
                          frame #0 {
                            # "Use first\naxis only."
                            # "Wait until move\nhas stopped or\nstop is pressed"
                            # "Move first axis 0.01 mm\nrelative to its current\nposition."
                            n65 = local read "Step Size (microns)"() -> (w296:dbl[])
                            n66 = Index Array(array=w302, index=0) -> (element=w305:string)
                            n67 = Build Array(w305) -> (w301:string[])
                            n68 = call "MOV.vi"("System no."=w297, "Axes to move"=w301, "Position values"=w296, "error in"=w311) -> ("error out"=w309:errorcluster)  [unwired: 1 in, 14 out]
                            n69 = call "General wait for movement to stop.vi"("System no."=w297, "Axes to wait for"=w301, "error in"=w309) -> ("error out"=w303:errorcluster)  [unwired: 5 in, 11 out]
                            n70 = call "POS?.vi"("System no."=w297, "Axes to query"=w301, "All axes?"=TRUE, "error in"=w303) -> ("Position"=w300:dbl[], "error out"=w308:errorcluster)  [unwired: 1 in, 13 out]
                            "Position" <- w300
                            n71 = Split 1D Array(array=w300, index=1) -> (first subarray=w298:dbl[])  [unwired: 1 out]
                            n72 = call "ERR?.vi"("System no."=w297, "error in"=w308) -> ("error out"=w307:errorcluster)  [unwired: 17 out]
                            n73 = Add Array Elements(numeric array=w298) -> ()  [unwired: 1 out]
                            n74 = call "GCSTranslateError.vi"("error in"=w307) -> ("error out"=w304:errorcluster)  [unwired: 18 out]
                          }
                          frame #1 {
                            n75 = global read "GlobalFramesToStr.vi" "Frames to Store"() -> (w324:u32)
                            n76 = call "ExSubCreateFile.vi"("error in (no error)"=w312, "Pulser Handle"=u32 0, "Camera Handle"=w313) -> ("error out"=w326:errorcluster, "Handles Out"=w322:T4)  [unwired: 1 in]
                            n77 = Unbundle(w322) -> ("File Handle"=w317:u32, "Image Handle"=w320:u32)  [unwired: 3 out]
                            n78 = call <userlib>:"CameraStart.vi"("error in"=w326) -> ("error out"=w321:errorcluster, "Camera Handle"=w319:u32)  [unwired: 1 in]
                            n79 = for {
                              N: w324 -> [_]
                              tunnel: w321 -> [w331]
                              tunnel: [w330] -> w323
                              tunnel: w317 -> [w329]
                              tunnel: w320 -> [w328]
                              tunnel: [w327] -> w316 mode=indexing
                              n80 = while {
                                tunnel: [w338] -> w330
                                tunnel: w331 -> [w336]
                                tunnel: w329 -> [w335]
                                tunnel: w328 -> [w334]
                                tunnel: [w333] -> w327
                                stop <- w339 stop-if-true
                                n81 = call <userlib>:"CameraCheckData.vi"("error in"=w336) -> ("Camera Handle"=w341:u32, "Number Of Frames Available"=w343:i32, "error out"=w340:errorcluster)  [unwired: 1 in]
                                n82 = Wait Until Next ms Multiple(millisecond multiple=u32 50) -> ()  [unwired: 1 out]
                                n83 = Greater Than 0?(x=w343) -> (x > 0?=w342:bool)
                                n84 = case shown="True" w342 {
                                selector: w342 -> [w344 w354]
                                tunnel: w341 -> [_ w356]
                                tunnel: w340 -> [w345 w355]
                                tunnel: [w344 w354] -> w339
                                tunnel: [w345 w349] -> w338
                                tunnel: w335 -> [_ w348]
                                tunnel: w334 -> [_ w347]
                                tunnel: [_ w346] -> w333
                                frame False {
                                }
                                frame True {
                                w350 = 1
                                n85 = call <userlib>:"CameraGetData.vi"("error in"=w355, "Image/Data Handle"=w347, "Camera Handle"=w356) -> ("error out"=w353:errorcluster, "Image/Data Handle"=w351:u32)  [unwired: 1 out]
                                n86 = call <userlib>:"FileSaveData.vi"("error in"=w353, "Image Handle"=w351, "File Handle"=w348) -> ("error out"=w352:errorcluster)  [unwired: 1 out]
                                n87 = call <userlib>:"ImageGetLineF32.vi"("error in"=w352, "Z Position"=w350, "Y Position"=w350, "Data Handle"=w351) -> ("error out"=w349:errorcluster, "Array F32"=w346:sgl[])  [unwired: 1 out]
                                }
                                }
                              }
                              n88 = Wait Until Next ms Multiple(millisecond multiple=u32 50) -> ()  [unwired: 1 out]
                            }
                            n89 = call <userlib>:"CameraStop.vi"("error in"=w323, "Camera Handle"=w319) -> ("error out"=w325:errorcluster, "Camera Handle"=w314:u32)
                            n90 = call "ExSubCloseFileImage.vi"("error in (no error)"=w325, "Handles In"=w322) -> ("error out"=w315:errorcluster)
                          }
                        }
                        n91 = Greater Or Equal?(x=w285, y="Number of Steps Down") -> (x >= y?=w290:bool)
                        n92 = Build Array (concatenate)(w277, w278) -> (w276:dbl[][])
                        n93 = Add Array Elements(numeric array=w278) -> (sum=w279:sgl)
                        n94 = Build Array(w279) -> (w295:sgl[])
                        n95 = Build Array (concatenate)(w294, w295) -> (w293:dbl[][])
                      }
                      n96 = call <vilib>:"Plot Helper.vi"("y matrix"=w272) -> ("2D Plotmatrix Class Obj Array out"=→"XY Plot Matrix":refnum<class "XY Plot Matrix Datatype.lvclass">[])  [unwired: 3 in, 7 out]
                    }
                    frame #1 {
                      # "Use first\naxis only."
                      # "Wait until move\nhas stopped or\nstop is pressed"
                      # "Move first axis 0.01 mm\nrelative to its current\nposition."
                      n97 = local read "Step Size (microns)"() -> (w358:dbl[])
                      n98 = Index Array(array=w364, index=1) -> (element=w369:string)
                      n99 = Build Array(w369) -> (w367:string[])
                      n100 = Absolute Value(x=w358) -> (abs(x)=w357:dbl[])
                      n101 = call "MOV.vi"("System no."=w361, "Axes to move"=w367, "Position values"=w357, "error in"=w363) -> ("error out"=w373:errorcluster)  [unwired: 1 in, 14 out]
                      n102 = call "General wait for movement to stop.vi"("System no."=w361, "Axes to wait for"=w367, "error in"=w373) -> ("error out"=w368:errorcluster)  [unwired: 5 in, 11 out]
                      n103 = call "POS?.vi"("System no."=w361, "Axes to query"=w367, "All axes?"=TRUE, "error in"=w368) -> ("Position"=w366:dbl[], "error out"=w372:errorcluster)  [unwired: 1 in, 13 out]
                      "Position 3" <- w366
                      n104 = Split 1D Array(array=w366, index=1) -> (second subarray=w359:dbl[])  [unwired: 1 out]
                      n105 = call "ERR?.vi"("System no."=w361, "error in"=w372) -> ("error out"=w371:errorcluster)  [unwired: 17 out]
                      n106 = call "GCSTranslateError.vi"("error in"=w371) -> ("error out"=w362:errorcluster)  [unwired: 18 out]
                      n107 = Split 1D Array(array=w359, index=1) -> ()  [unwired: 2 out]
                    }
                  }
                  n108 = Array To Spreadsheet String(array=w250, 3:"%f" ("format string")) -> (spreadsheet string=w252:string)  [unwired: 1 in]
                  "Line Number" <- w242
                }
                n109 = local read "Number of Steps Left"() -> (w218:dbl)
                n110 = local read "Exposure 2"() -> (w221:dbl)
                n111 = call <userlib>:"CameraShutter.vi"("Camera Handle"=w233, "error in"=w231) -> ("Camera Handle"=w232:u32, "error out"=w230:errorcluster)  [unwired: 3 in]
                n112 = call "File Dialog3"("start path"=path "C:/Users/Raman Lab/Desktop/Molly") -> ("selected path"=w234:path)  [unwired: 11 in, 3 out]
                n113 = local read "Number of Steps Down"() -> (w226:dbl)
                n114 = Number To Decimal String(number=w218) -> (decimal integer string=w217:string)  [unwired: 1 in]
                n115 = Number To Fractional String(number=w226) -> (F-format string=w225:string)  [unwired: 3 in]
                n116 = Number To Decimal String(number=w221) -> (decimal integer string=w222:string)  [unwired: 1 in]
                n117 = Concatenate Strings(w225, "\r\n", w217, "\r\n", w222, "\r\n", w227) -> (w236:string)
                n118 = Write to Text File(file (use dialog)=w234, text=w236) -> ()  [unwired: 2 in, 3 out]
              }
            }
          }
        }
      }
      frame "Stage Control" {
        n119 = case shown="True" "?" {
          tunnel: w375 -> [_ w417]
          tunnel: w376 -> [_ w416]
          frame False {
          }
          frame True {
            n120 = stacked-sequence {
              seq-local: [w419 _] -> [_ w439]
              seq-local: [w418 _] -> [_ w438]
              tunnel: w416 -> [w420 _]
              tunnel: w417 -> [w421 _]
              frame #0 {
                n121 = stacked-sequence {
                  tunnel: w421 -> [w425]
                  tunnel: w420 -> [w424]
                  tunnel: [w423] -> w418
                  tunnel: [w422] -> w419
                  frame #0 {
                    w437 = cluster{"S/N":string, "USB Search?":bool} {"S/N"="", "USB Search?"=TRUE}  # USB settings
                    w433 = u16 2 items=["RS232", "TCP/IP", "USB"] ("Interface")
                    w432 = cluster{"Portnumber":i32, "Baudrate":u16} {"Portnumber"=0, "Baudrate"=5}  # RS232 settings
                    w431 = T3 {"Host address/name"="", "Port"=50000, "Board"=0, "TCP/IP Search?"=TRUE}  # TCP/IP settings
                    # "TRUE: We want to\nmove the axis to its middle\nposition"
                    # "System number is one"
                    n122 = call "E727_Configuration_Setup.vi"("System no."=w424, "USB settings"=w437, "Are stages connected?"=bool[] [TRUE, TRUE, FALSE], "Change servo status to ON?"=TRUE ("Use dialog to define\nconnected stages?"), "Perform autozero?"=FALSE ("Use dialog to define\nconnected stages?"), "error in"=w425, "Interface"=w433, "RS232 settings"=w432, "TCP/IP settings"=w431, "Stop wave generator\noutput (if any)"=TRUE ("All axes?"), "Move to middle?"=FALSE) -> ("All conn. axes"=w422:string[], "error out"=w427:errorcluster)  [unwired: 3 in, 4 out]
                    n123 = call "POS?.vi"("System no."=w424, "Axes to query"=w422, "All axes?"=TRUE, "error in"=w427) -> ("Position"=→"Position 4":dbl[], "error out"=w423:errorcluster)  [unwired: 1 in, 13 out]
                  }
                }
              }
              frame #1 {
                n124 = stacked-sequence {
                  tunnel: w439 -> [w442]
                  tunnel: w438 -> [w441]
                  frame #0 {
                    w440 = 1
                    # "Use first\naxis only."
                    # "Wait until move\nhas stopped or\nstop is pressed"
                    # "Move first axis 0.01 mm\nrelative to its current\nposition."
                    n125 = local read "Step Size (microns) Y"() -> (w443:dbl[])
                    n126 = Index Array(array=w442, index=0) -> (element=w447:string)
                    n127 = Build Array(w447) -> (w445:string[])
                    n128 = call "MOV.vi"("System no."=w440, "Axes to move"=w445, "Position values"=w443, "error in"=w441) -> ("error out"=w451:errorcluster)  [unwired: 1 in, 14 out]
                    n129 = call "General wait for movement to stop.vi"("System no."=w440, "Axes to wait for"=w445, "error in"=w451) -> ("error out"=w446:errorcluster)  [unwired: 5 in, 11 out]
                    n130 = call "POS?.vi"("System no."=w440, "Axes to query"=w445, "All axes?"=TRUE, "error in"=w446) -> ("Position"=→"Position 5":dbl[], "error out"=w450:errorcluster)  [unwired: 1 in, 13 out]
                    n131 = call "ERR?.vi"("System no."=w440, "error in"=w450) -> ("error out"=w449:errorcluster)  [unwired: 17 out]
                    n132 = call "GCSTranslateError.vi"("error in"=w449) -> ()  [unwired: 19 out]
                  }
                }
              }
            }
          }
        }
        n133 = case shown="True" "?" {
          tunnel: w375 -> [_ w380]
          tunnel: w376 -> [_ w379]
          frame False {
          }
          frame True {
            n134 = stacked-sequence {
              seq-local: [w382 _] -> [_ w402]
              seq-local: [w381 _] -> [_ w401]
              tunnel: w379 -> [w383 _]
              tunnel: w380 -> [w384 _]
              frame #0 {
                n135 = stacked-sequence {
                  tunnel: w384 -> [w388]
                  tunnel: w383 -> [w387]
                  tunnel: [w386] -> w381
                  tunnel: [w385] -> w382
                  frame #0 {
                    w400 = cluster{"S/N":string, "USB Search?":bool} {"S/N"="", "USB Search?"=TRUE}  # USB settings
                    w396 = u16 2 items=["RS232", "TCP/IP", "USB"] ("Interface")
                    w395 = cluster{"Portnumber":i32, "Baudrate":u16} {"Portnumber"=0, "Baudrate"=5}  # RS232 settings
                    w394 = T3 {"Host address/name"="", "Port"=50000, "Board"=0, "TCP/IP Search?"=TRUE}  # TCP/IP settings
                    # "TRUE: We want to\nmove the axis to its middle\nposition"
                    # "System number is one"
                    n136 = call "E727_Configuration_Setup.vi"("System no."=w387, "USB settings"=w400, "Are stages connected?"=bool[] [TRUE, TRUE, FALSE], "Change servo status to ON?"=TRUE ("Use dialog to define\nconnected stages?"), "Perform autozero?"=FALSE ("Use dialog to define\nconnected stages?"), "error in"=w388, "Interface"=w396, "RS232 settings"=w395, "TCP/IP settings"=w394, "Stop wave generator\noutput (if any)"=TRUE ("All axes?"), "Move to middle?"=FALSE) -> ("All conn. axes"=w385:string[], "error out"=w390:errorcluster)  [unwired: 3 in, 4 out]
                    n137 = call "POS?.vi"("System no."=w387, "Axes to query"=w385, "All axes?"=TRUE, "error in"=w390) -> ("Position"=→"Position 7":dbl[], "error out"=w386:errorcluster)  [unwired: 1 in, 13 out]
                  }
                }
              }
              frame #1 {
                n138 = stacked-sequence {
                  tunnel: w402 -> [w405]
                  tunnel: w401 -> [w404]
                  frame #0 {
                    w403 = 1
                    # "Use first\naxis only."
                    # "Wait until move\nhas stopped or\nstop is pressed"
                    # "Move first axis 0.01 mm\nrelative to its current\nposition."
                    n139 = local read "Step Size (microns) X"() -> (w406:dbl[])
                    n140 = Index Array(array=w405, index=1) -> (element=w410:string)
                    n141 = Build Array(w410) -> (w408:string[])
                    n142 = call "MOV.vi"("System no."=w403, "Axes to move"=w408, "Position values"=w406, "error in"=w404) -> ("error out"=w414:errorcluster)  [unwired: 1 in, 14 out]
                    n143 = call "General wait for movement to stop.vi"("System no."=w403, "Axes to wait for"=w408, "error in"=w414) -> ("error out"=w409:errorcluster)  [unwired: 5 in, 11 out]
                    n144 = call "POS?.vi"("System no."=w403, "Axes to query"=w408, "All axes?"=TRUE, "error in"=w409) -> ("Position"=→"Position 8":dbl[], "error out"=w413:errorcluster)  [unwired: 1 in, 13 out]
                    n145 = call "ERR?.vi"("System no."=w403, "error in"=w413) -> ("error out"=w412:errorcluster)  [unwired: 17 out]
                    n146 = call "GCSTranslateError.vi"("error in"=w412) -> ()  [unwired: 19 out]
                  }
                }
              }
            }
          }
        }
      }
    }
    n147 = global read "GlobalCamOpen.vi" "Camera Opened"() -> (w23:u32)
    n148 = Not(x="Release Camera") -> (.not. x?=w16:bool)
    n149 = Greater Than 0?(x=w23) -> (x > 0?=w22:bool)
    n150 = And(x=w16, y=w22) -> (x .and. y?=→"Camera Opened":bool)
    n151 = Wait Until Next ms Multiple(millisecond multiple=5) -> ()  [unwired: 1 out]
  }
  n152 = call <userlib>:"CameraClose.vi"("error in"=w8, "Camera Handle"=w5) -> ("error out"=w7:errorcluster)
  n153 = call "Close connection if open.vi"("System no."=w1) -> ("error out"=→"error out 2":errorcluster)  [unwired: 2 in, 16 out]
  n154 = call <userlib>:"UninitToolkit.vi"("error in"=w7) -> ("error out"=→"error out":errorcluster)
